vi "FipsAdjacent.vi"() -> (11 "Fips":i32[](array[numeric]))   [LabVIEW 2017] (continued)
Parish, LA\"\t22019\n\"Calcasieu Parish, LA\"\t22019\t\"Cameron Parish, LA\"\t22023\n\"Calcasieu Parish, LA\"\t22019\t\"Jefferson Davis Parish, LA\"\t22053\n\"Calcasieu Parish, LA\"\t22019\t\"Newton County, TX\"\t48351\n\"Calcasieu Parish, LA\"\t22019\t\"Orange County, TX\"\t48361\n\"Caldwell Parish, LA\"\t22021\t\"Caldwell Parish, LA\"\t22021\n\"Caldwell Parish, LA\"\t22021\t\"Catahoula Parish, LA\"\t22025\n\"Caldwell Parish, LA\"\t22021\t\"Franklin Parish, LA\"\t22041\n\"Caldwell Parish, LA\"\t22021\t\"Jackson Parish, LA\"\t22049\n\"Caldwell Parish, LA\"\t22021\t\"La Salle Parish, LA\"\t22059\n\"Caldwell Parish, LA\"\t22021\t\"Ouachita Parish, LA\"\t22073\n\"Caldwell Parish, LA\"\t22021\t\"Richland Parish, LA\"\t22083\n\"Caldwell Parish, LA\"\t22021\t\"Winn Parish, LA\"\t22127\n\"Cameron Parish, LA\"\t22023\t\"Calcasieu Parish, LA\"\t22019\n\"Cameron Parish, LA\"\t22023\t\"Cameron Parish, LA\"\t22023\n\"Cameron Parish, LA\"\t22023\t\"Jefferson Davis Parish, LA\"\t22053\n\"Cameron Parish, LA\"\t22023\t\"Vermilion Parish, LA\"\t22113\n\"Cameron Parish, LA\"\t22023\t\"Jefferson County, TX\"\t48245\n\"Cameron Parish, LA\"\t22023\t\"Orange County, TX\"\t48361\n\"Catahoula Parish, LA\"\t22025\t\"Avoyelles Parish, LA\"\t22009\n\"Catahoula Parish, LA\"\t22025\t\"Caldwell Parish, LA\"\t22021\n\"Catahoula Parish, LA\"\t22025\t\"Catahoula Parish, LA\"\t22025\n\"Catahoula Parish, LA\"\t22025\t\"Concordia Parish, LA\"\t22029\n\"Catahoula Parish, LA\"\t22025\t\"Franklin Parish, LA\"\t22041\n\"Catahoula Parish, LA\"\t22025\t\"La Salle Parish, LA\"\t22059\n\"Catahoula Parish, LA\"\t22025\t\"Tensas Parish, LA\"\t22107\n\"Claiborne Parish, LA\"\t22027\t\"Columbia County, AR\"\t05027\n\"Claiborne Parish, LA\"\t22027\t\"Union County, AR\"\t05139\n\"Claiborne Parish, LA\"\t22027\t\"Bienville Parish, LA\"\t22013\n\"Claiborne Parish, LA\"\t22027\t\"Claiborne Parish, LA\"\t22027\n\"Claiborne Parish, LA\"\t22027\t\"Lincoln Parish, LA\"\t22061\n\"Claiborne Parish, LA\"\t22027\t\"Union Parish, LA\"\t22111\n\"Claiborne Parish, LA\"\t22027\t\"Webster Parish, LA\"\t22119\n\"Concordia Parish, LA\"\t22029\t\"Avoyelles Parish, LA\"\t22009\n\"Concordia Parish, LA\"\t22029\t\"Catahoula Parish, LA\"\t22025\n\"Concordia Parish, LA\"\t22029\t\"Concordia Parish, LA\"\t22029\n\"Concordia Parish, LA\"\t22029\t\"Pointe Coupee Parish, LA\"\t22077\n\"Concordia Parish, LA\"\t22029\t\"Tensas Parish, LA\"\t22107\n\"Concordia Parish, LA\"\t22029\t\"West Feliciana Parish, LA\"\t22125\n\"Concordia Parish, LA\"\t22029\t\"Adams County, MS\"\t28001\n\"Concordia Parish, LA\"\t22029\t\"Wilkinson County, MS\"\t28157\n\"De Soto Parish, LA\"\t22031\t\"Caddo Parish, LA\"\t22017\n\"De Soto Parish, LA\"\t22031\t\"De Soto Parish, LA\"\t22031\n\"De Soto Parish, LA\"\t22031\t\"Natchitoches Parish, LA\"\t22069\n\"De Soto Parish, LA\"\t22031\t\"Red River Parish, LA\"\t22081\n\"De Soto Parish, LA\"\t22031\t\"Sabine Parish, LA\"\t22085\n\"De Soto Parish, LA\"\t22031\t\"Panola County, TX\"\t48365\n\"De Soto Parish, LA\"\t22031\t\"Shelby County, TX\"\t48419\n\"East Baton Rouge Parish, LA\"\t22033\t\"Ascension Parish, LA\"\t22005\n\"East Baton Rouge Parish, LA\"\t22033\t\"East Baton Rouge Parish, LA\"\t22033\n\"East Baton Rouge Parish, LA\"\t22033\t\"East Feliciana Parish, LA\"\t22037\n\"East Baton Rouge Parish, LA\"\t22033\t\"Iberville Parish, LA\"\t22047\n\"East Baton Rouge Parish, LA\"\t22033\t\"Livingston Parish, LA\"\t22063\n\"East Baton Rouge Parish, LA\"\t22033\t\"St. Helena Parish, LA\"\t22091\n\"East Baton Rouge Parish, LA\"\t22033\t\"West Baton Rouge Parish, LA\"\t22121\n\"East Carroll Parish, LA\"\t22035\t\"Chicot County, AR\"\t05017\n\"East Carroll Parish, LA\"\t22035\t\"East Carroll Parish, LA\"\t22035\n\"East Carroll Parish, LA\"\t22035\t\"Madison Parish, LA\"\t22065\n\"East Carroll Parish, LA\"\t22035\t\"Richland Parish, LA\"\t22083\n\"East Carroll Parish, LA\"\t22035\t\"West Carroll Parish, LA\"\t22123\n\"East Carroll Parish, LA\"\t22035\t\"Issaquena County, MS\"\t28055\n\"East Carroll Parish, LA\"\t22035\t\"Warren County, MS\"\t28149\n\"East Feliciana Parish, LA\"\t22037\t\"East Baton Rouge Parish, LA\"\t22033\n\"East Feliciana Parish, LA\"\t22037\t\"East Feliciana Parish, LA\"\t22037\n\"East Feliciana Parish, LA\"\t22037\t\"St. Helena Parish, LA\"\t22091\n\"East Feliciana Parish, LA\"\t22037\t\"West Baton Rouge Parish, LA\"\t22121\n\"East Feliciana Parish, LA\"\t22037\t\"West Feliciana Parish, LA\"\t22125\n\"East Feliciana Parish, LA\"\t22037\t\"Amite County, MS\"\t28005\n\"East Feliciana Parish, LA\"\t22037\t\"Wilkinson County, MS\"\t28157\n\"Evangeline Parish, LA\"\t22039\t\"Acadia Parish, LA\"\t22001\n\"Evangeline Parish, LA\"\t22039\t\"Allen Parish, LA\"\t22003\n\"Evangeline Parish, LA\"\t22039\t\"Avoyelles Parish, LA\"\t22009\n\"Evangeline Parish, LA\"\t22039\t\"Evangeline Parish, LA\"\t22039\n\"Evangeline Parish, LA\"\t22039\t\"Jefferson Davis Parish, LA\"\t22053\n\"Evangeline Parish, LA\"\t22039\t\"Rapides Parish, LA\"\t22079\n\"Evangeline Parish, LA\"\t22039\t\"St. Landry Parish, LA\"\t22097\n\"Franklin Parish, LA\"\t22041\t\"Caldwell Parish, LA\"\t22021\n\"Franklin Parish, LA\"\t22041\t\"Catahoula Parish, LA\"\t22025\n\"Franklin Parish, LA\"\t22041\t\"Franklin Parish, LA\"\t22041\n\"Franklin Parish, LA\"\t22041\t\"Madison Parish, LA\"\t22065\n\"Franklin Parish, LA\"\t22041\t\"Richland Parish, LA\"\t22083\n\"Franklin Parish, LA\"\t22041\t\"Tensas Parish, LA\"\t22107\n\"Grant Parish, LA\"\t22043\t\"Grant Parish, LA\"\t22043\n\"Grant Parish, LA\"\t22043\t\"La Salle Parish, LA\"\t22059\n\"Grant Parish, LA\"\t22043\t\"Natchitoches Parish, LA\"\t22069\n\"Grant Parish, LA\"\t22043\t\"Rapides Parish, LA\"\t22079\n\"Grant Parish, LA\"\t22043\t\"Winn Parish, LA\"\t22127\n\"Iberia Parish, LA\"\t22045\t\"Assumption Parish, LA\"\t22007\n\"Iberia Parish, LA\"\t22045\t\"Iberia Parish, LA\"\t22045\n\"Iberia Parish, LA\"\t22045\t\"Iberville Parish, LA\"\t22047\n\"Iberia Parish, LA\"\t22045\t\"Lafayette Parish, LA\"\t22055\n\"Iberia Parish, LA\"\t22045\t\"St. Martin Parish, LA\"\t22099\n\"Iberia Parish, LA\"\t22045\t\"St. Mary Parish, LA\"\t22101\n\"Iberia Parish, LA\"\t22045\t\"Vermilion Parish, LA\"\t22113\n\"Iberville Parish, LA\"\t22047\t\"Ascension Parish, LA\"\t22005\n\"Iberville Parish, LA\"\t22047\t\"Assumption Parish, LA\"\t22007\n\"Iberville Parish, LA\"\t22047\t\"East Baton Rouge Parish, LA\"\t22033\n\"Iberville Parish, LA\"\t22047\t\"Iberia Parish, LA\"\t22045\n\"Iberville Parish, LA\"\t22047\t\"Iberville Parish, LA\"\t22047\n\"Iberville Parish, LA\"\t22047\t\"Pointe Coupee Parish, LA\"\t22077\n\"Iberville Parish, LA\"\t22047\t\"St. Martin Parish, LA\"\t22099\n\"Iberville Parish, LA\"\t22047\t\"West Baton Rouge Parish, LA\"\t22121\n\"Jackson Parish, LA\"\t22049\t\"Bienville Parish, LA\"\t22013\n\"Jackson Parish, LA\"\t22049\t\"Caldwell Parish, LA\"\t22021\n\"Jackson Parish, LA\"\t22049\t\"Jackson Parish, LA\"\t22049\n\"Jackson Parish, LA\"\t22049\t\"Lincoln Parish, LA\"\t22061\n\"Jackson Parish, LA\"\t22049\t\"Ouachita Parish, LA\"\t22073\n\"Jackson Parish, LA\"\t22049\t\"Winn Parish, LA\"\t22127\n\"Jefferson Parish, LA\"\t22051\t\"Jefferson Parish, LA\"\t22051\n\"Jefferson Parish, LA\"\t22051\t\"Lafourche Parish, LA\"\t22057\n\"Jefferson Parish, LA\"\t22051\t\"Orleans Parish, LA\"\t22071\n\"Jefferson Parish, LA\"\t22051\t\"Plaquemines Parish, LA\"\t22075\n\"Jefferson Parish, LA\"\t22051\t\"St. Charles Parish, LA\"\t22089\n\"Jefferson Parish, LA\"\t22051\t\"St. John the Baptist Parish, LA\"\t22095\n\"Jefferson Parish, LA\"\t22051\t\"St. Tammany Parish, LA\"\t22103\n\"Jefferson Parish, LA\"\t22051\t\"Tangipahoa Parish, LA\"\t22105\n\"Jefferson Davis Parish, LA\"\t22053\t\"Acadia Parish, LA\"\t22001\n\"Jefferson Davis Parish, LA\"\t22053\t\"Allen Parish, LA\"\t22003\n\"Jefferson Davis Parish, LA\"\t22053\t\"Beauregard Parish, LA\"\t22011\n\"Jefferson Davis Parish, LA\"\t22053\t\"Calcasieu Parish, LA\"\t22019\n\"Jefferson Davis Parish, LA\"\t22053\t\"Cameron Parish, LA\"\t22023\n\"Jefferson Davis Parish, LA\"\t22053\t\"Evangeline Parish, LA\"\t22039\n\"Jefferson Davis Parish, LA\"\t22053\t\"Jefferson Davis Parish, LA\"\t22053\n\"Jefferson Davis Parish, LA\"\t22053\t\"Vermilion Parish, LA\"\t22113\n\"Lafayette Parish, LA\"\t22055\t\"Acadia Parish, LA\"\t22001\n\"Lafayette Parish, LA\"\t22055\t\"Iberia Parish, LA\"\t22045\n\"Lafayette Parish, LA\"\t22055\t\"Lafayette Parish, LA\"\t22055\n\"Lafayette Parish, LA\"\t22055\t\"St. Landry Parish, LA\"\t22097\n\"Lafayette Parish, LA\"\t22055\t\"St. Martin Parish, LA\"\t22099\n\"Lafayette Parish, LA\"\t22055\t\"Vermilion Parish, LA\"\t22113\n\"Lafourche Parish, LA\"\t22057\t\"Assumption Parish, LA\"\t22007\n\"Lafourche Parish, LA\"\t22057\t\"Jefferson Parish, LA\"\t22051\n\"Lafourche Parish, LA\"\t22057\t\"Lafourche Parish, LA\"\t22057\n\"Lafourche Parish, LA\"\t22057\t\"St. Charles Parish, LA\"\t22089\n\"Lafourche Parish, LA\"\t22057\t\"St. James Parish, LA\"\t22093\n\"Lafourche Parish, LA\"\t22057\t\"St. John the Baptist Parish, LA\"\t22095\n\"Lafourche Parish, LA\"\t22057\t\"Terrebonne Parish, LA\"\t22109\n\"La Salle Parish, LA\"\t22059\t\"Avoyelles Parish, LA\"\t22009\n\"La Salle Parish, LA\"\t22059\t\"Caldwell Parish, LA\"\t22021\n\"La Salle Parish, LA\"\t22059\t\"Catahoula Parish, LA\"\t22025\n\"La Salle Parish, LA\"\t22059\t\"Grant Parish, LA\"\t22043\n\"La Salle Parish, LA\"\t22059\t\"La Salle Parish, LA\"\t22059\n\"La Salle Parish, LA\"\t22059\t\"Rapides Parish, LA\"\t22079\n\"La Salle Parish, LA\"\t22059\t\"Winn Parish, LA\"\t22127\n\"Lincoln Parish, LA\"\t22061\t\"Bienville Parish, LA\"\t22013\n\"Lincoln Parish, LA\"\t22061\t\"Claiborne Parish, LA\"\t22027\n\"Lincoln Parish, LA\"\t22061\t\"Jackson Parish, LA\"\t22049\n\"Lincoln Parish, LA\"\t22061\t\"Lincoln Parish, LA\"\t22061\n\"Lincoln Parish, LA\"\t22061\t\"Ouachita Parish, LA\"\t22073\n\"Lincoln Parish, LA\"\t22061\t\"Union Parish, LA\"\t22111\n\"Livingston Parish, LA\"\t22063\t\"Ascension Parish, LA\"\t22005\n\"Livingston Parish, LA\"\t22063\t\"East Baton Rouge Parish, LA\"\t22033\n\"Livingston Parish, LA\"\t22063\t\"Livingston Parish, LA\"\t22063\n\"Livingston Parish, LA\"\t22063\t\"St. Helena Parish, LA\"\t22091\n\"Livingston Parish, LA\"\t22063\t\"St. John the Baptist Parish, LA\"\t22095\n\"Livingston Parish, LA\"\t22063\t\"Tangipahoa Parish, LA\"\t22105\n\"Madison Parish, LA\"\t22065\t\"East Carroll Parish, LA\"\t22035\n\"Madison Parish, LA\"\t22065\t\"Franklin Parish, LA\"\t22041\n\"Madison Parish, LA\"\t22065\t\"Madison Parish, LA\"\t22065\n\"Madison Parish, LA\"\t22065\t\"Richland Parish, LA\"\t22083\n\"Madison Parish, LA\"\t22065\t\"Tensas Parish, LA\"\t22107\n\"Madison Parish, LA\"\t22065\t\"Warren County, MS\"\t28149\n\"Morehouse Parish, LA\"\t22067\t\"Ashley County, AR\"\t05003\n\"Morehouse Parish, LA\"\t22067\t\"Chicot County, AR\"\t05017\n\"Morehouse Parish, LA\"\t22067\t\"Union County, AR\"\t05139\n\"Morehouse Parish, LA\"\t22067\t\"Morehouse Parish, LA\"\t22067\n\"Morehouse Parish, LA\"\t22067\t\"Ouachita Parish, LA\"\t22073\n\"Morehouse Parish, LA\"\t22067\t\"Richland Parish, LA\"\t22083\n\"Morehouse Parish, LA\"\t22067\t\"Union Parish, LA\"\t22111\n\"Morehouse Parish, LA\"\t22067\t\"West Carroll Parish, LA\"\t22123\n\"Natchitoches Parish, LA\"\t22069\t\"Bienville Parish, LA\"\t22013\n\"Natchitoches Parish, LA\"\t22069\t\"De Soto Parish, LA\"\t22031\n\"Natchitoches Parish, LA\"\t22069\t\"Grant Parish, LA\"\t22043\n\"Natchitoches Parish, LA\"\t22069\t\"Natchitoches Parish, LA\"\t22069\n\"Natchitoches Parish, LA\"\t22069\t\"Rapides Parish, LA\"\t22079\n\"Natchitoches Parish, LA\"\t22069\t\"Red River Parish, LA\"\t22081\n\"Natchitoches Parish, LA\"\t22069\t\"Sabine Parish, LA\"\t22085\n\"Natchitoches Parish, LA\"\t22069\t\"Vernon Parish, LA\"\t22115\n\"Natchitoches Parish, LA\"\t22069\t\"Winn Parish, LA\"\t22127\n\"Orleans Parish, LA\"\t22071\t\"Jefferson Parish, LA\"\t22051\n\"Orleans Parish, LA\"\t22071\t\"Orleans Parish, LA\"\t22071\n\"Orleans Parish, LA\"\t22071\t\"Plaquemines Parish, LA\"\t22075\n\"Orleans Parish, LA\"\t22071\t\"St. Bernard Parish, LA\"\t22087\n\"Orleans Parish, LA\"\t22071\t\"St. Tammany Parish, LA\"\t22103\n\"Ouachita Parish, LA\"\t22073\t\"Caldwell Parish, LA\"\t22021\n\"Ouachita Parish, LA\"\t22073\t\"Jackson Parish, LA\"\t22049\n\"Ouachita Parish, LA\"\t22073\t\"Lincoln Parish, LA\"\t22061\n\"Ouachita Parish, LA\"\t22073\t\"Morehouse Parish, LA\"\t22067\n\"Ouachita Parish, LA\"\t22073\t\"Ouachita Parish, LA\"\t22073\n\"Ouachita Parish, LA\"\t22073\t\"Richland Parish, LA\"\t22083\n\"Ouachita Parish, LA\"\t22073\t\"Union Parish, LA\"\t22111\n\"Plaquemines Parish, LA\"\t22075\t\"Jefferson Parish, LA\"\t22051\n\"Plaquemines Parish, LA\"\t22075\t\"Orleans Parish, LA\"\t22071\n\"Plaquemines Parish, LA\"\t22075\t\"Plaquemines Parish, LA\"\t22075\n\"Plaquemines Parish, LA\"\t22075\t\"St. Bernard Parish, LA\"\t22087\n\"Pointe Coupee Parish, LA\"\t22077\t\"Avoyelles Parish, LA\"\t22009\n\"Pointe Coupee Parish, LA\"\t22077\t\"Concordia Parish, LA\"\t22029\n\"Pointe Coupee Parish, LA\"\t22077\t\"Iberville Parish, LA\"\t22047\n\"Pointe Coupee Parish, LA\"\t22077\t\"Pointe Coupee Parish, LA\"\t22077\n\"Pointe Coupee Parish, LA\"\t22077\t\"St. Landry Parish, LA\"\t22097\n\"Pointe Coupee Parish, LA\"\t22077\t\"St. Martin Parish, LA\"\t22099\n\"Pointe Coupee Parish, LA\"\t22077\t\"West Baton Rouge Parish, LA\"\t22121\n\"Pointe Coupee Parish, LA\"\t22077\t\"West Feliciana Parish, LA\"\t22125\n\"Rapides Parish, LA\"\t22079\t\"Allen Parish, LA\"\t22003\n\"Rapides Parish, LA\"\t22079\t\"Avoyelles Parish, LA\"\t22009\n\"Rapides Parish, LA\"\t22079\t\"Evangeline Parish, LA\"\t22039\n\"Rapides Parish, LA\"\t22079\t\"Grant Parish, LA\"\t22043\n\"Rapides Parish, LA\"\t22079\t\"La Salle Parish, LA\"\t22059\n\"Rapides Parish, LA\"\t22079\t\"Natchitoches Parish, LA\"\t22069\n\"Rapides Parish, LA\"\t22079\t\"Rapides Parish, LA\"\t22079\n\"Rapides Parish, LA\"\t22079\t\"Vernon Parish, LA\"\t22115\n\"Red River Parish, LA\"\t22081\t\"Bienville Parish, LA\"\t22013\n\"Red River Parish, LA\"\t22081\t\"Bossier Parish, LA\"\t22015\n\"Red River Parish, LA\"\t22081\t\"Caddo Parish, LA\"\t22017\n\"Red River Parish, LA\"\t22081\t\"De Soto Parish, LA\"\t22031\n\"Red River Parish, LA\"\t22081\t\"Natchitoches Parish, LA\"\t22069\n\"Red River Parish, LA\"\t22081\t\"Red River Parish, LA\"\t22081\n\"Richland Parish, LA\"\t22083\t\"Caldwell Parish, LA\"\t22021\n\"Richland Parish, LA\"\t22083\t\"East Carroll Parish, LA\"\t22035\n\"Richland Parish, LA\"\t22083\t\"Franklin Parish, LA\"\t22041\n\"Richland Parish, LA\"\t22083\t\"Madison Parish, LA\"\t22065\n\"Richland Parish, LA\"\t22083\t\"Morehouse Parish, LA\"\t22067\n\"Richland Parish, LA\"\t22083\t\"Ouachita Parish, LA\"\t22073\n\"Richland Parish, LA\"\t22083\t\"Richland Parish, LA\"\t22083\n\"Richland Parish, LA\"\t22083\t\"West Carroll Parish, LA\"\t22123\n\"Sabine Parish, LA\"\t22085\t\"De Soto Parish, LA\"\t22031\n\"Sabine Parish, LA\"\t22085\t\"Natchitoches Parish, LA\"\t22069\n\"Sabine Parish, LA\"\t22085\t\"Sabine Parish, LA\"\t22085\n\"Sabine Parish, LA\"\t22085\t\"Vernon Parish, LA\"\t22115\n\"Sabine Parish, LA\"\t22085\t\"Newton County, TX\"\t48351\n\"Sabine Parish, LA\"\t22085\t\"Sabine County, TX\"\t48403\n\"Sabine Parish, LA\"\t22085\t\"Shelby County, TX\"\t48419\n\"St. Bernard Parish, LA\"\t22087\t\"Orleans Parish, LA\"\t22071\n\"St. Bernard Parish, LA\"\t22087\t\"Plaquemines Parish, LA\"\t22075\n\"St. Bernard Parish, LA\"\t22087\t\"St. Bernard Parish, LA\"\t22087\n\"St. Bernard Parish, LA\"\t22087\t\"St. Tammany Parish, LA\"\t22103\n\"St. Bernard Parish, LA\"\t22087\t\"Hancock County, MS\"\t28045\n\"St. Bernard Parish, LA\"\t22087\t\"Harrison County, MS\"\t28047\n\"St. Charles Parish, LA\"\t22089\t\"Jefferson Parish, LA\"\t22051\n\"St. Charles Parish, LA\"\t22089\t\"Lafourche Parish, LA\"\t22057\n\"St. Charles Parish, LA\"\t22089\t\"St. Charles Parish, LA\"\t22089\n\"St. Charles Parish, LA\"\t22089\t\"St. John the Baptist Parish, LA\"\t22095\n\"St. Charles Parish, LA\"\t22089\t\"Tangipahoa Parish, LA\"\t22105\n\"St. Helena Parish, LA\"\t22091\t\"East Baton Rouge Parish, LA\"\t22033\n\"St. Helena Parish, LA\"\t22091\t\"East Feliciana Parish, LA\"\t22037\n\"St. Helena Parish, LA\"\t22091\t\"Livingston Parish, LA\"\t22063\n\"St. Helena Parish, LA\"\t22091\t\"St. Helena Parish, LA\"\t22091\n\"St. Helena Parish, LA\"\t22091\t\"Tangipahoa Parish, LA\"\t22105\n\"St. Helena Parish, LA\"\t22091\t\"Amite County, MS\"\t28005\n\"St. James Parish, LA\"\t22093\t\"Ascension Parish, LA\"\t22005\n\"St. James Parish, LA\"\t22093\t\"Assumption Parish, LA\"\t22007\n\"St. James Parish, LA\"\t22093\t\"Lafourche Parish, LA\"\t22057\n\"St. James Parish, LA\"\t22093\t\"St. James Parish, LA\"\t22093\n\"St. James Parish, LA\"\t22093\t\"St. John the Baptist Parish, LA\"\t22095\n\"St. John the Baptist Parish, LA\"\t22095\t\"Ascension Parish, LA\"\t22005\n\"St. John the Baptist Parish, LA\"\t22095\t\"Jefferson Parish, LA\"\t22051\n\"St. John the Baptist Parish, LA\"\t22095\t\"Lafourche Parish, LA\"\t22057\n\"St. John the Baptist Parish, LA\"\t22095\t\"Livingston Parish, LA\"\t22063\n\"St. John the Baptist Parish, LA\"\t22095\t\"St. Charles Parish, LA\"\t22089\n\"St. John the Baptist Parish, LA\"\t22095\t\"St. James Parish, LA\"\t22093\n\"St. John the Baptist Parish, LA\"\t22095\t\"St. John the Baptist Parish, LA\"\t22095\n\"St. John the Baptist Parish, LA\"\t22095\t\"Tangipahoa Parish, LA\"\t22105\n\"St. Landry Parish, LA\"\t22097\t\"Acadia Parish, LA\"\t22001\n\"St. Landry Parish, LA\"\t22097\t\"Avoyelles Parish, LA\"\t22009\n\"St. Landry Parish, LA\"\t22097\t\"Evangeline Parish, LA\"\t22039\n\"St. Landry Parish, LA\"\t22097\t\"Lafayette Parish, LA\"\t22055\n\"St. Landry Parish, LA\"\t22097\t\"Pointe Coupee Parish, LA\"\t22077\n\"St. Landry Parish, LA\"\t22097\t\"St. Landry Parish, LA\"\t22097\n\"St. Landry Parish, LA\"\t22097\t\"St. Martin Parish, LA\"\t22099\n\"St. Martin Parish, LA\"\t22099\t\"Assumption Parish, LA\"\t22007\n\"St. Martin Parish, LA\"\t22099\t\"Iberia Parish, LA\"\t22045\n\"St. Martin Parish, LA\"\t22099\t\"Iberville Parish, LA\"\t22047\n\"St. Martin Parish, LA\"\t22099\t\"Lafayette Parish, LA\"\t22055\n\"St. Martin Parish, LA\"\t22099\t\"Pointe Coupee Parish, LA\"\t22077\n\"St. Martin Parish, LA\"\t22099\t\"St. Landry Parish, LA\"\t22097\n\"St. Martin Parish, LA\"\t22099\t\"St. Martin Parish, LA\"\t22099\n\"St. Martin Parish, LA\"\t22099\t\"St. Mary Parish, LA\"\t22101\n\"St. Mary Parish, LA\"\t22101\t\"Assumption Parish, LA\"\t22007\n\"St. Mary Parish, LA\"\t22101\t\"Iberia Parish, LA\"\t22045\n\"St. Mary Parish, LA\"\t22101\t\"St. Martin Parish, LA\"\t22099\n\"St. Mary Parish, LA\"\t22101\t\"St. Mary Parish, LA\"\t22101\n\"St. Mary Parish, LA\"\t22101\t\"Terrebonne Parish, LA\"\t22109\n\"St. Tammany Parish, LA\"\t22103\t\"Jefferson Parish, LA\"\t22051\n\"St. Tammany Parish, LA\"\t22103\t\"Orleans Parish, LA\"\t22071\n\"St. Tammany Parish, LA\"\t22103\t\"St. Bernard Parish, LA\"\t22087\n\"St. Tammany Parish, LA\"\t22103\t\"St. Tammany Parish, LA\"\t22103\n\"St. Tammany Parish, LA\"\t22103\t\"Tangipahoa Parish, LA\"\t22105\n\"St. Tammany Parish, LA\"\t22103\t\"Washington Parish, LA\"\t22117\n\"St. Tammany Parish, LA\"\t22103\t\"Hancock County, MS\"\t28045\n\"St. Tammany Parish, LA\"\t22103\t\"Pearl River County, MS\"\t28109\n\"Tangipahoa Parish, LA\"\t22105\t\"Jefferson Parish, LA\"\t22051\n\"Tangipahoa Parish, LA\"\t22105\t\"Livingston Parish, LA\"\t22063\n\"Tangipahoa Parish, LA\"\t22105\t\"St. Charles Parish, LA\"\t22089\n\"Tangipahoa Parish, LA\"\t22105\t\"St. Helena Parish, LA\"\t22091\n\"Tangipahoa Parish, LA\"\t22105\t\"St. John the Baptist Parish, LA\"\t22095\n\"Tangipahoa Parish, LA\"\t22105\t\"St. Tammany Parish, LA\"\t22103\n\"Tangipahoa Parish, LA\"\t22105\t\"Tangipahoa Parish, LA\"\t22105\n\"Tangipahoa Parish, LA\"\t22105\t\"Washington Parish, LA\"\t22117\n\"Tangipahoa Parish, LA\"\t22105\t\"Amite County, MS\"\t28005\n\"Tangipahoa Parish, LA\"\t22105\t\"Pike County, MS\"\t28113\n\"Tensas Parish, LA\"\t22107\t\"Catahoula Parish, LA\"\t22025\n\"Tensas Parish, LA\"\t22107\t\"Concordia Parish, LA\"\t22029\n\"Tensas Parish, LA\"\t22107\t\"Franklin Parish, LA\"\t22041\n\"Tensas Parish, LA\"\t22107\t\"Madison Parish, LA\"\t22065\n\"Tensas Parish, LA\"\t22107\t\"Tensas Parish, LA\"\t22107\n\"Tensas Parish, LA\"\t22107\t\"Adams County, MS\"\t28001\n\"Tensas Parish, LA\"\t22107\t\"Claiborne County, MS\"\t28021\n\"Tensas Parish, LA\"\t22107\t\"Jefferson County, MS\"\t28063\n\"Tensas Parish, LA\"\t22107\t\"Warren County, MS\"\t28149\n\"Terrebonne Parish, LA\"\t22109\t\"Assumption Parish, LA\"\t22007\n\"Terrebonne Parish, LA\"\t22109\t\"Lafourche Parish, LA\"\t22057\n\"Terrebonne Parish, LA\"\t22109\t\"St. Mary Parish, LA\"\t22101\n\"Terrebonne Parish, LA\"\t22109\t\"Terrebonne Parish, LA\"\t22109\n\"Union Parish, LA\"\t22111\t\"Ashley County, AR\"\t05003\n\"Union Parish, LA\"\t22111\t\"Union County, AR\"\t05139\n\"Union Parish, LA\"\t22111\t\"Claiborne Parish, LA\"\t22027\n\"Union Parish, LA\"\t22111\t\"Lincoln Parish, LA\"\t22061\n\"Union Parish, LA\"\t22111\t\"Morehouse Parish, LA\"\t22067\n\"Union Parish, LA\"\t22111\t\"Ouachita Parish, LA\"\t22073\n\"Union Parish, LA\"\t22111\t\"Union Parish, LA\"\t22111\n\"Vermilion Parish, LA\"\t22113\t\"Acadia Parish, LA\"\t22001\n\"Vermilion Parish, LA\"\t22113\t\"Cameron Parish, LA\"\t22023\n\"Vermilion Parish, LA\"\t22113\t\"Iberia Parish, LA\"\t22045\n\"Vermilion Parish, LA\"\t22113\t\"Jefferson Davis Parish, LA\"\t22053\n\"Vermilion Parish, LA\"\t22113\t\"Lafayette Parish, LA\"\t22055\n\"Vermilion Parish, LA\"\t22113\t\"Vermilion Parish, LA\"\t22113\n\"Vernon Parish, LA\"\t22115\t\"Allen Parish, LA\"\t22003\n\"Vernon Parish, LA\"\t22115\t\"Beauregard Parish, LA\"\t22011\n\"Vernon Parish, LA\"\t22115\t\"Natchitoches Parish, LA\"\t22069\n\"Vernon Parish, LA\"\t22115\t\"Rapides Parish, LA\"\t22079\n\"Vernon Parish, LA\"\t22115\t\"Sabine Parish, LA\"\t22085\n\"Vernon Parish, LA\"\t22115\t\"Vernon Parish, LA\"\t22115\n\"Vernon Parish, LA\"\t22115\t\"Newton County, TX\"\t48351\n\"Washington Parish, LA\"\t22117\t\"St. Tammany Parish, LA\"\t22103\n\"Washington Parish, LA\"\t22117\t\"Tangipahoa Parish, LA\"\t22105\n\"Washington Parish, LA\"\t22117\t\"Washington Parish, LA\"\t22117\n\"Washington Parish, LA\"\t22117\t\"Marion County, MS\"\t28091\n\"Washington Parish, LA\"\t22117\t\"Pearl River County, MS\"\t28109\n\"Washington Parish, LA\"\t22117\t\"Pike County, MS\"\t28113\n\"Washington Parish, LA\"\t22117\t\"Walthall County, MS\"\t28147\n\"Webster Parish, LA\"\t22119\t\"Columbia County, AR\"\t05027\n\"Webster Parish, LA\"\t22119\t\"Lafayette County, AR\"\t05073\n\"Webster Parish, LA\"\t22119\t\"Bienville Parish, LA\"\t22013\n\"Webster Parish, LA\"\t22119\t\"Bossier Parish, LA\"\t22015\n\"Webster Parish, LA\"\t22119\t\"Claiborne Parish, LA\"\t22027\n\"Webster Parish, LA\"\t22119\t\"Webster Parish, LA\"\t22119\n\"West Baton Rouge Parish, LA\"\t22121\t\"East Baton Rouge Parish, LA\"\t22033\n\"West Baton Rouge Parish, LA\"\t22121\t\"East Feliciana Parish, LA\"\t22037\n\"West Baton Rouge Parish, LA\"\t22121\t\"Iberville Parish, LA\"\t22047\n\"West Baton Rouge Parish, LA\"\t22121\t\"Pointe Coupee Parish, LA\"\t22077\n\"West Baton Rouge Parish, LA\"\t22121\t\"West Baton Rouge Parish, LA\"\t22121\n\"West Baton Rouge Parish, LA\"\t22121\t\"West Feliciana Parish, LA\"\t22125\n\"West Carroll Parish, LA\"\t22123\t\"Chicot County, AR\"\t05017\n\"West Carroll Parish, LA\"\t22123\t\"East Carroll Parish, LA\"\t22035\n\"West Carroll Parish, LA\"\t22123\t\"Morehouse Parish, LA\"\t22067\n\"West Carroll Parish, LA\"\t22123\t\"Richland Parish, LA\"\t22083\n\"West Carroll Parish, LA\"\t22123\t\"West Carroll Parish, LA\"\t22123\n\"West Feliciana Parish, LA\"\t22125\t\"Avoyelles Parish, LA\"\t22009\n\"West Feliciana Parish, LA\"\t22125\t\"Concordia Parish, LA\"\t22029\n\"West Feliciana Parish, LA\"\t22125\t\"East Feliciana Parish, LA\"\t22037\n\"West Feliciana Parish, LA\"\t22125\t\"Pointe Coupee Parish, LA\"\t22077\n\"West Feliciana Parish, LA\"\t22125\t\"West Baton Rouge Parish, LA\"\t22121\n\"West Feliciana Parish, LA\"\t22125\t\"West Feliciana Parish, LA\"\t22125\n\"West Feliciana Parish, LA\"\t22125\t\"Wilkinson County, MS\"\t28157\n\"Winn Parish, LA\"\t22127\t\"Bienville Parish, LA\"\t22013\n\"Winn Parish, LA\"\t22127\t\"Caldwell Parish, LA\"\t22021\n\"Winn Parish, LA\"\t22127\t\"Grant Parish, LA\"\t22043\n\"Winn Parish, LA\"\t22127\t\"Jackson Parish, LA\"\t22049\n\"Winn Parish, LA\"\t22127\t\"La Salle Parish, LA\"\t22059\n\"Winn Parish, LA\"\t22127\t\"Natchitoches Parish, LA\"\t22069\n\"Winn Parish, LA\"\t22127\t\"Winn Parish, LA\"\t22127\n\"Androscoggin County, ME\"\t23001\t\"Androscoggin County, ME\"\t23001\n\"Androscoggin County, ME\"\t23001\t\"Cumberland County, ME\"\t23005\n\"Androscoggin County, ME\"\t23001\t\"Franklin County, ME\"\t23007\n\"Androscoggin County, ME\"\t23001\t\"Kennebec County, ME\"\t23011\n\"Androscoggin County, ME\"\t23001\t\"Oxford County, ME\"\t23017\n\"Androscoggin County, ME\"\t23001\t\"Sagadahoc County, ME\"\t23023\n\"Aroostook County, ME\"\t23003\t\"Aroostook County, ME\"\t23003\n\"Aroostook County, ME\"\t23003\t\"Penobscot County, ME\"\t23019\n\"Aroostook County, ME\"\t23003\t\"Piscataquis County, ME\"\t23021\n\"Aroostook County, ME\"\t23003\t\"Somerset County, ME\"\t23025\n\"Aroostook County, ME\"\t23003\t\"Washington County, ME\"\t23029\n\"Cumberland County, ME\"\t23005\t\"Androscoggin County, ME\"\t23001\n\"Cumberland County, ME\"\t23005\t\"Cumberland County, ME\"\t23005\n\"Cumberland County, ME\"\t23005\t\"Oxford County, ME\"\t23017\n\"Cumberland County, ME\"\t23005\t\"Sagadahoc County, ME\"\t23023\n\"Cumberland County, ME\"\t23005\t\"York County, ME\"\t23031\n\"Franklin County, ME\"\t23007\t\"Androscoggin County, ME\"\t23001\n\"Franklin County, ME\"\t23007\t\"Franklin County, ME\"\t23007\n\"Franklin County, ME\"\t23007\t\"Kennebec County, ME\"\t23011\n\"Franklin County, ME\"\t23007\t\"Oxford County, ME\"\t23017\n\"Franklin County, ME\"\t23007\t\"Somerset County, ME\"\t23025\n\"Hancock County, ME\"\t23009\t\"Hancock County, ME\"\t23009\n\"Hancock County, ME\"\t23009\t\"Knox County, ME\"\t23013\n\"Hancock County, ME\"\t23009\t\"Penobscot County, ME\"\t23019\n\"Hancock County, ME\"\t23009\t\"Waldo County, ME\"\t23027\n\"Hancock County, ME\"\t23009\t\"Washington County, ME\"\t23029\n\"Kennebec County, ME\"\t23011\t\"Androscoggin County, ME\"\t23001\n\"Kennebec County, ME\"\t23011\t\"Franklin County, ME\"\t23007\n\"Kennebec County, ME\"\t23011\t\"Kennebec County, ME\"\t23011\n\"Kennebec County, ME\"\t23011\t\"Lincoln County, ME\"\t23015\n\"Kennebec County, ME\"\t23011\t\"Sagadahoc County, ME\"\t23023\n\"Kennebec County, ME\"\t23011\t\"Somerset County, ME\"\t23025\n\"Kennebec County, ME\"\t23011\t\"Waldo County, ME\"\t23027\n\"Knox County, ME\"\t23013\t\"Hancock County, ME\"\t23009\n\"Knox County, ME\"\t23013\t\"Knox County, ME\"\t23013\n\"Knox County, ME\"\t23013\t\"Lincoln County, ME\"\t23015\n\"Knox County, ME\"\t23013\t\"Waldo County, ME\"\t23027\n\"Lincoln County, ME\"\t23015\t\"Kennebec County, ME\"\t23011\n\"Lincoln County, ME\"\t23015\t\"Knox County, ME\"\t23013\n\"Lincoln County, ME\"\t23015\t\"Lincoln County, ME\"\t23015\n\"Lincoln County, ME\"\t23015\t\"Sagadahoc County, ME\"\t23023\n\"Lincoln County, ME\"\t23015\t\"Waldo County, ME\"\t23027\n\"Oxford County, ME\"\t23017\t\"Androscoggin County, ME\"\t23001\n\"Oxford County, ME\"\t23017\t\"Cumberland County, ME\"\t23005\n\"Oxford County, ME\"\t23017\t\"Franklin County, ME\"\t23007\n\"Oxford County, ME\"\t23017\t\"Oxford County, ME\"\t23017\n\"Oxford County, ME\"\t23017\t\"York County, ME\"\t23031\n\"Oxford County, ME\"\t23017\t\"Carroll County, NH\"\t33003\n\"Oxford County, ME\"\t23017\t\"Coos County, NH\"\t33007\n\"Penobscot County, ME\"\t23019\t\"Aroostook County, ME\"\t23003\n\"Penobscot County, ME\"\t23019\t\"Hancock County, ME\"\t23009\n\"Penobscot County, ME\"\t23019\t\"Penobscot County, ME\"\t23019\n\"Penobscot County, ME\"\t23019\t\"Piscataquis County, ME\"\t23021\n\"Penobscot County, ME\"\t23019\t\"Somerset County, ME\"\t23025\n\"Penobscot County, ME\"\t23019\t\"Waldo County, ME\"\t23027\n\"Penobscot County, ME\"\t23019\t\"Washington County, ME\"\t23029\n\"Piscataquis County, ME\"\t23021\t\"Aroostook County, ME\"\t23003\n\"Piscataquis County, ME\"\t23021\t\"Penobscot County, ME\"\t23019\n\"Piscataquis County, ME\"\t23021\t\"Piscataquis County, ME\"\t23021\n\"Piscataquis County, ME\"\t23021\t\"Somerset County, ME\"\t23025\n\"Sagadahoc County, ME\"\t23023\t\"Androscoggin County, ME\"\t23001\n\"Sagadahoc County, ME\"\t23023\t\"Cumberland County, ME\"\t23005\n\"Sagadahoc County, ME\"\t23023\t\"Kennebec County, ME\"\t23011\n\"Sagadahoc County, ME\"\t23023\t\"Lincoln County, ME\"\t23015\n\"Sagadahoc County, ME\"\t23023\t\"Sagadahoc County, ME\"\t23023\n\"Somerset County, ME\"\t23025\t\"Aroostook County, ME\"\t23003\n\"Somerset County, ME\"\t23025\t\"Franklin County, ME\"\t23007\n\"Somerset County, ME\"\t23025\t\"Kennebec County, ME\"\t23011\n\"Somerset County, ME\"\t23025\t\"Penobscot County, ME\"\t23019\n\"Somerset County, ME\"\t23025\t\"Piscataquis County, ME\"\t23021\n\"Somerset County, ME\"\t23025\t\"Somerset County, ME\"\t23025\n\"Somerset County, ME\"\t23025\t\"Waldo County, ME\"\t23027\n\"Waldo County, ME\"\t23027\t\"Hancock County, ME\"\t23009\n\"Waldo County, ME\"\t23027\t\"Kennebec County, ME\"\t23011\n\"Waldo County, ME\"\t23027\t\"Knox County, ME\"\t23013\n\"Waldo County, ME\"\t23027\t\"Lincoln County, ME\"\t23015\n\"Waldo County, ME\"\t23027\t\"Penobscot County, ME\"\t23019\n\"Waldo County, ME\"\t23027\t\"Somerset County, ME\"\t23025\n\"Waldo County, ME\"\t23027\t\"Waldo County, ME\"\t23027\n\"Washington County, ME\"\t23029\t\"Aroostook County, ME\"\t23003\n\"Washington County, ME\"\t23029\t\"Hancock County, ME\"\t23009\n\"Washington County, ME\"\t23029\t\"Penobscot County, ME\"\t23019\n\"Washington County, ME\"\t23029\t\"Washington County, ME\"\t23029\n\"York County, ME\"\t23031\t\"Cumberland County, ME\"\t23005\n\"York County, ME\"\t23031\t\"Oxford County, ME\"\t23017\n\"York County, ME\"\t23031\t\"York County, ME\"\t23031\n\"York County, ME\"\t23031\t\"Carroll County, NH\"\t33003\n\"York County, ME\"\t23031\t\"Rockingham County, NH\"\t33015\n\"York County, ME\"\t23031\t\"Strafford County, NH\"\t33017\n\"Allegany County, MD\"\t24001\t\"Allegany County, MD\"\t24001\n\"Allegany County, MD\"\t24001\t\"Garrett County, MD\"\t24023\n\"Allegany County, MD\"\t24001\t\"Washington County, MD\"\t24043\n\"Allegany County, MD\"\t24001\t\"Bedford County, PA\"\t42009\n\"Allegany County, MD\"\t24001\t\"Fulton County, PA\"\t42057\n\"Allegany County, MD\"\t24001\t\"Somerset County, PA\"\t42111\n\"Allegany County, MD\"\t24001\t\"Hampshire County, WV\"\t54027\n\"Allegany County, MD\"\t24001\t\"Mineral County, WV\"\t54057\n\"Allegany County, MD\"\t24001\t\"Morgan County, WV\"\t54065\n\"Anne Arundel County, MD\"\t24003\t\"Anne Arundel County, MD\"\t24003\n\"Anne Arundel County, MD\"\t24003\t\"Baltimore County, MD\"\t24005\n\"Anne Arundel County, MD\"\t24003\t\"Calvert County, MD\"\t24009\n\"Anne Arundel County, MD\"\t24003\t\"Howard County, MD\"\t24027\n\"Anne Arundel County, MD\"\t24003\t\"Kent County, MD\"\t24029\n\"Anne Arundel County, MD\"\t24003\t\"Prince George's County, MD\"\t24033\n\"Anne Arundel County, MD\"\t24003\t\"Queen Anne's County, MD\"\t24035\n\"Anne Arundel County, MD\"\t24003\t\"Talbot County, MD\"\t24041\n\"Anne Arundel County, MD\"\t24003\t\"Baltimore city, MD\"\t24510\n\"Baltimore County, MD\"\t24005\t\"Anne Arundel County, MD\"\t24003\n\"Baltimore County, MD\"\t24005\t\"Baltimore County, MD\"\t24005\n\"Baltimore County, MD\"\t24005\t\"Carroll County, MD\"\t24013\n\"Baltimore County, MD\"\t24005\t\"Harford County, MD\"\t24025\n\"Baltimore County, MD\"\t24005\t\"Howard County, MD\"\t24027\n\"Baltimore County, MD\"\t24005\t\"Kent County, MD\"\t24029\n\"Baltimore County, MD\"\t24005\t\"Baltimore city, MD\"\t24510\n\"Baltimore County, MD\"\t24005\t\"York County, PA\"\t42133\n\"Calvert County, MD\"\t24009\t\"Anne Arundel County, MD\"\t24003\n\"Calvert County, MD\"\t24009\t\"Calvert County, MD\"\t24009\n\"Calvert County, MD\"\t24009\t\"Charles County, MD\"\t24017\n\"Calvert County, MD\"\t24009\t\"Dorchester County, MD\"\t24019\n\"Calvert County, MD\"\t24009\t\"Prince George's County, MD\"\t24033\n\"Calvert County, MD\"\t24009\t\"St. Mary's County, MD\"\t24037\n\"Calvert County, MD\"\t24009\t\"Talbot County, MD\"\t24041\n\"Caroline County, MD\"\t24011\t\"Kent County, DE\"\t10001\n\"Caroline County, MD\"\t24011\t\"Sussex County, DE\"\t10005\n\"Caroline County, MD\"\t24011\t\"Caroline County, MD\"\t24011\n\"Caroline County, MD\"\t24011\t\"Dorchester County, MD\"\t24019\n\"Caroline County, MD\"\t24011\t\"Queen Anne's County, MD\"\t24035\n\"Caroline County, MD\"\t24011\t\"Talbot County, MD\"\t24041\n\"Carroll County, MD\"\t24013\t\"Baltimore County, MD\"\t24005\n\"Carroll County, MD\"\t24013\t\"Carroll County, MD\"\t24013\n\"Carroll County, MD\"\t24013\t\"Frederick County, MD\"\t24021\n\"Carroll County, MD\"\t24013\t\"Howard County, MD\"\t24027\n\"Carroll County, MD\"\t24013\t\"Adams County, PA\"\t42001\n\"Carroll County, MD\"\t24013\t\"York County, PA\"\t42133\n\"Cecil County, MD\"\t24015\t\"New Castle County, DE\"\t10003\n\"Cecil County, MD\"\t24015\t\"Cecil County, MD\"\t24015\n\"Cecil County, MD\"\t24015\t\"Harford County, MD\"\t24025\n\"Cecil County, MD\"\t24015\t\"Kent County, MD\"\t24029\n\"Cecil County, MD\"\t24015\t\"Chester County, PA\"\t42029\n\"Cecil County, MD\"\t24015\t\"Lancaster County, PA\"\t42071\n\"Charles County, MD\"\t24017\t\"Calvert County, MD\"\t24009\n\"Charles County, MD\"\t24017\t\"Charles County, MD\"\t24017\n\"Charles County, MD\"\t24017\t\"Prince George's County, MD\"\t24033\n\"Charles County, MD\"\t24017\t\"St. Mary's County, MD\"\t24037\n\"Charles County, MD\"\t24017\t\"Fairfax County, VA\"\t51059\n\"Charles County, MD\"\t24017\t\"King George County, VA\"\t51099\n\"Charles County, MD\"\t24017\t\"Prince William County, VA\"\t51153\n\"Charles County, MD\"\t24017\t\"Stafford County, VA\"\t51179\n\"Charles County, MD\"\t24017\t\"Westmoreland County, VA\"\t51193\n\"Dorchester County, MD\"\t24019\t\"Sussex County, DE\"\t10005\n\"Dorchester County, MD\"\t24019\t\"Calvert County, MD\"\t24009\n\"Dorchester County, MD\"\t24019\t\"Caroline County, MD\"\t24011\n\"Dorchester County, MD\"\t24019\t\"Dorchester County, MD\"\t24019\n\"Dorchester County, MD\"\t24019\t\"St. Mary's County, MD\"\t24037\n\"Dorchester County, MD\"\t24019\t\"Somerset County, MD\"\t24039\n\"Dorchester County, MD\"\t24019\t\"Talbot County, MD\"\t24041\n\"Dorchester County, MD\"\t24019\t\"Wicomico County, MD\"\t24045\n\"Frederick County, MD\"\t24021\t\"Carroll County, MD\"\t24013\n\"Frederick County, MD\"\t24021\t\"Frederick County, MD\"\t24021\n\"Frederick County, MD\"\t24021\t\"Howard County, MD\"\t24027\n\"Frederick County, MD\"\t24021\t\"Montgomery County, MD\"\t24031\n\"Frederick County, MD\"\t24021\t\"Washington County, MD\"\t24043\n\"Frederick County, MD\"\t24021\t\"Adams County, PA\"\t42001\n\"Frederick County, MD\"\t24021\t\"Franklin County, PA\"\t42055\n\"Frederick County, MD\"\t24021\t\"Loudoun County, VA\"\t51107\n\"Garrett County, MD\"\t24023\t\"Allegany County, MD\"\t24001\n\"Garrett County, MD\"\t24023\t\"Garrett County, MD\"\t24023\n\"Garrett County, MD\"\t24023\t\"Fayette County, PA\"\t42051\n\"Garrett County, MD\"\t24023\t\"Somerset County, PA\"\t42111\n\"Garrett County, MD\"\t24023\t\"Grant County, WV\"\t54023\n\"Garrett County, MD\"\t24023\t\"Mineral County, WV\"\t54057\n\"Garrett County, MD\"\t24023\t\"Preston County, WV\"\t54077\n\"Harford County, MD\"\t24025\t\"Baltimore County, MD\"\t24005\n\"Harford County, MD\"\t24025\t\"Cecil County, MD\"\t24015\n\"Harford County, MD\"\t24025\t\"Harford County, MD\"\t24025\n\"Harford County, MD\"\t24025\t\"Kent County, MD\"\t24029\n\"Harford County, MD\"\t24025\t\"Lancaster County, PA\"\t42071\n\"Harford County, MD\"\t24025\t\"York County, PA\"\t42133\n\"Howard County, MD\"\t24027\t\"Anne Arundel County, MD\"\t24003\n\"Howard County, MD\"\t24027\t\"Baltimore County, MD\"\t24005\n\"Howard County, MD\"\t24027\t\"Carroll County, MD\"\t24013\n\"Howard County, MD\"\t24027\t\"Frederick County, MD\"\t24021\n\"Howard County, MD\"\t24027\t\"Howard County, MD\"\t24027\n\"Howard County, MD\"\t24027\t\"Montgomery County, MD\"\t24031\n\"Howard County, MD\"\t24027\t\"Prince George's County, MD\"\t24033\n\"Kent County, MD\"\t24029\t\"Kent County, DE\"\t10001\n\"Kent County, MD\"\t24029\t\"New Castle County, DE\"\t10003\n\"Kent County, MD\"\t24029\t\"Anne Arundel County, MD\"\t24003\n\"Kent County, MD\"\t24029\t\"Baltimore County, MD\"\t24005\n\"Kent County, MD\"\t24029\t\"Cecil County, MD\"\t24015\n\"Kent County, MD\"\t24029\t\"Harford County, MD\"\t24025\n\"Kent County, MD\"\t24029\t\"Kent County, MD\"\t24029\n\"Kent County, MD\"\t24029\t\"Queen Anne's County, MD\"\t24035\n\"Montgomery County, MD\"\t24031\t\"District of Columbia, DC\"\t11001\n\"Montgomery County, MD\"\t24031\t\"Frederick County, MD\"\t24021\n\"Montgomery County, MD\"\t24031\t\"Howard County, MD\"\t24027\n\"Montgomery County, MD\"\t24031\t\"Montgomery County, MD\"\t24031\n\"Montgomery County, MD\"\t24031\t\"Prince George's County, MD\"\t24033\n\"Montgomery County, MD\"\t24031\t\"Arlington County, VA\"\t51013\n\"Montgomery County, MD\"\t24031\t\"Fairfax County, VA\"\t51059\n\"Montgomery County, MD\"\t24031\t\"Loudoun County, VA\"\t51107\n\"Prince George's County, MD\"\t24033\t\"District of Columbia, DC\"\t11001\n\"Prince George's County, MD\"\t24033\t\"Anne Arundel County, MD\"\t24003\n\"Prince George's County, MD\"\t24033\t\"Calvert County, MD\"\t24009\n\"Prince George's County, MD\"\t24033\t\"Charles County, MD\"\t24017\n\"Prince George's County, MD\"\t24033\t\"Howard County, MD\"\t24027\n\"Prince George's County, MD\"\t24033\t\"Montgomery County, MD\"\t24031\n\"Prince George's County, MD\"\t24033\t\"Prince George's County, MD\"\t24033\n\"Prince George's County, MD\"\t24033\t\"Fairfax County, VA\"\t51059\n\"Prince George's County, MD\"\t24033\t\"Alexandria city, VA\"\t51510\n\"Queen Anne's County, MD\"\t24035\t\"Kent County, DE\"\t10001\n\"Queen Anne's County, MD\"\t24035\t\"Anne Arundel County, MD\"\t24003\n\"Queen Anne's County, MD\"\t24035\t\"Caroline County, MD\"\t24011\n\"Queen Anne's County, MD\"\t24035\t\"Kent County, MD\"\t24029\n\"Queen Anne's County, MD\"\t24035\t\"Queen Anne's County, MD\"\t24035\n\"Queen Anne's County, MD\"\t24035\t\"Talbot County, MD\"\t24041\n\"St. Mary's County, MD\"\t24037\t\"Calvert County, MD\"\t24009\n\"St. Mary's County, MD\"\t24037\t\"Charles County, MD\"\t24017\n\"St. Mary's County, MD\"\t24037\t\"Dorchester County, MD\"\t24019\n\"St. Mary's County, MD\"\t24037\t\"St. Mary's County, MD\"\t24037\n\"St. Mary's County, MD\"\t24037\t\"Somerset County, MD\"\t24039\n\"St. Mary's County, MD\"\t24037\t\"Northumberland County, VA\"\t51133\n\"St. Mary's County, MD\"\t24037\t\"Westmoreland County, VA\"\t51193\n\"Somerset County, MD\"\t24039\t\"Dorchester County, MD\"\t24019\n\"Somerset County, MD\"\t24039\t\"St. Mary's County, MD\"\t24037\n\"Somerset County, MD\"\t24039\t\"Somerset County, MD\"\t24039\n\"Somerset County, MD\"\t24039\t\"Wicomico County, MD\"\t24045\n\"Somerset County, MD\"\t24039\t\"Worcester County, MD\"\t24047\n\"Somerset County, MD\"\t24039\t\"Accomack County, VA\"\t51001\n\"Somerset County, MD\"\t24039\t\"Northumberland County, VA\"\t51133\n\"Talbot County, MD\"\t24041\t\"Anne Arundel County, MD\"\t24003\n\"Talbot County, MD\"\t24041\t\"Calvert County, MD\"\t24009\n\"Talbot County, MD\"\t24041\t\"Caroline County, MD\"\t24011\n\"Talbot County, MD\"\t24041\t\"Dorchester County, MD\"\t24019\n\"Talbot County, MD\"\t24041\t\"Queen Anne's County, MD\"\t24035\n\"Talbot County, MD\"\t24041\t\"Talbot County, MD\"\t24041\n\"Washington County, MD\"\t24043\t\"Allegany County, MD\"\t24001\n\"Washington County, MD\"\t24043\t\"Frederick County, MD\"\t24021\n\"Washington 
